vi "RTM CreateFramesSection.vi"(8 "error in (no error)":errorcluster, 10 "Frame":string="Tx FRAME ", 11 "Node Ptr":T1 format="%.0x") -> (0 "error out":errorcluster, 3 "Node Ptr 2":T1 format="%.0x")   [LabVIEW 2018, in "CAN Gateway System Explorer.lvlib"]
uses:
  CAN Gateway System Explorer.lvlib
  <vilib>/NI Veristand/Custom Device API/Custom Device Item Ref.ctl
  Types/FramesCluster.ctl
  <vilib>/NI Veristand/Custom Device API/Get Item Property (Variant).vi
  Shared/Constants.vi
  <vilib>/NI Veristand/Custom Device Tools/Custom Device Utility Library/NI VeriStand - Search for Item by Name.vi
  <vilib>/NI Veristand/Custom Device API/Custom Device API.lvlib
  Shared/CAN Gateway Shared.lvlib
  <vilib>/NI Veristand/Custom Device Tools/Custom Device Utility Library/Custom Device Utility Library.lvlib
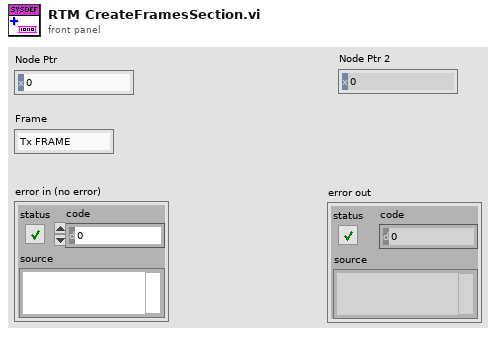
[diagram p1: front panel]
types:
  T1 = typedef "Custom Device API.lvlib/Custom Device Item Ref.ctl" = u64
  T2 = typedef "CAN Gateway System Explorer.lvlib/FramesCluster.ctl" = cluster{"Frame":string, "Fault":bool}
  T3 = typedef "Custom Device API.lvlib/Custom Device Item Info.ctl" = cluster{"Name":string, "Is Channel":bool, "GUID":string, "Is Waveform":bool}
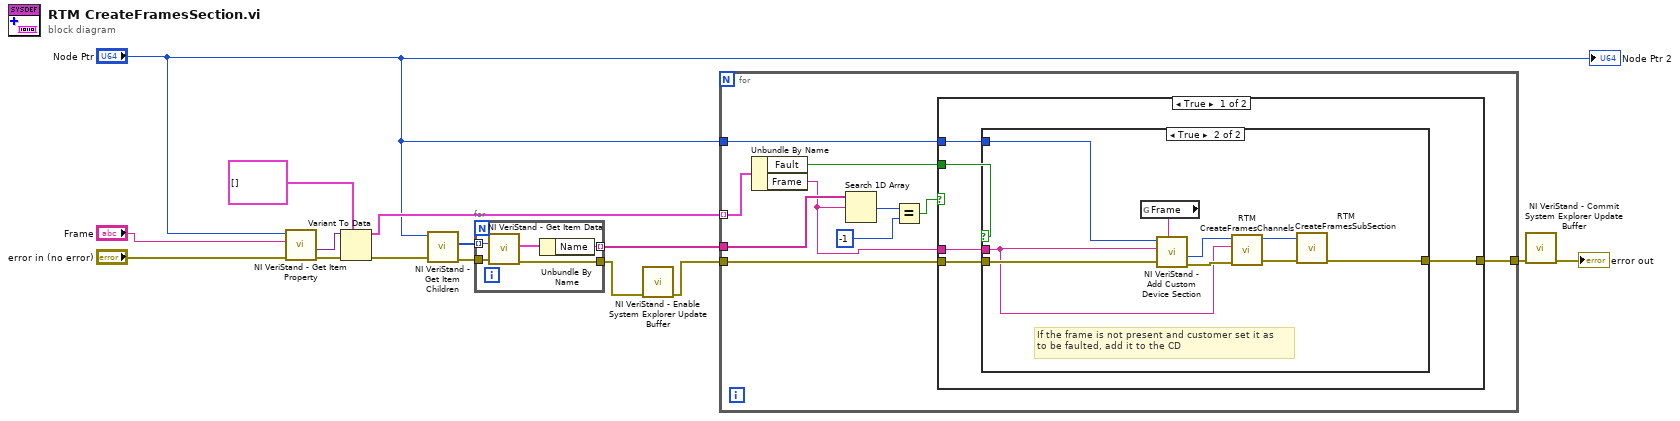
[diagram p0: block diagram]
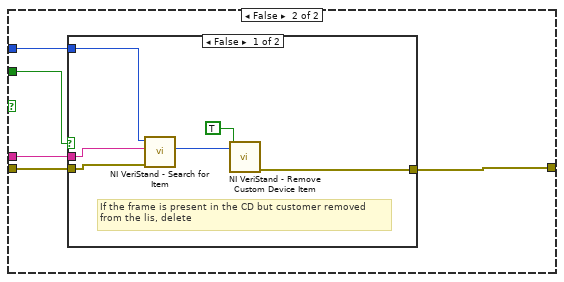
[diagram p3: hidden frame]
diagram:
  n1 = call-poly <vilib>:"NI VeriStand - Get Item Property.vi"("error in (no error)"="error in (no error)", "Property Name"="Frame", "Item Ref in"="Node Ptr") -> ("error out"=w14:errorcluster, "Value"=w15:variant)  [unwired: 5 in, 2 out]
  n2 = Variant To Data(error in=w14, type=T2[] [], Variant=w15) -> (data=w10:T2[], error out=w11:errorcluster)
  n3 = call <vilib>:"NI VeriStand - Get Item Children.vi"("error in (no error)"=w11, "Item Ref in"="Node Ptr") -> ("error out"=w7:errorcluster, "Child Refs"=w9:T1[])  [unwired: 6 in, 2 out]
  n4 = for {
    tunnel: w9 -> [w20] mode=indexing
    tunnel: [w18] -> w8 mode=indexing
    tunnel: w7 -> [w17]
    tunnel: [w16] -> w5
    n5 = call <vilib>:"NI VeriStand - Get Item Data.vi"("error in (no error)"=w17, "Item Ref in"=w20) -> ("error out"=w16:errorcluster, "Item Info"=w19:T3)  [unwired: 6 in, 2 out]
    n6 = Unbundle By Name(w19) -> ("Name"=w18:string)
  }
  n7 = call <vilib>:"NI VeriStand - Enable System Explorer Update Buffer.vi"("error in (no error)"=w5) -> ("error out"=w4:errorcluster)  [unwired: 10 in]
  n8 = for {
    tunnel: w10 -> [w30] mode=indexing
    tunnel: w8 -> [w29]
    tunnel: w4 -> [w26]
    tunnel: [w25] -> w3
    tunnel: "Node Ptr" -> [w21]
    n9 = Unbundle By Name(w30) -> ("Fault"=w23:bool, "Frame"=w22:string)
    n10 = Search 1D Array(1D array=w29, element=w22) -> (index of element=w27:i32)  [unwired: 1 in]
    n11 = Equal?(x=w27, y=-1 ("x")) -> (x = y?=w24:bool)
    n12 = case shown="True" w24 {
      tunnel: w26 -> [w35 w50]
      tunnel: [w34 w49] -> w25
      tunnel: w23 -> [w31 w46]
      tunnel: w22 -> [w33 w48]
      tunnel: w21 -> [w32 w47]
      frame True {
        n13 = case shown="True" w31 {
          tunnel: w35 -> [w36 w45]
          tunnel: [w36 w37] -> w34
          tunnel: w33 -> [_ w40]
          tunnel: w32 -> [_ w44]
          frame False {
          }
          frame True {
            # "If the frame is not present and customer set it as \nto be faulted, add it to the CD"
            n14 = global read "Constants.vi" "Frame"() -> (w43:string)
            n15 = call <vilib>:"NI VeriStand - Add Custom Device Section.vi"("GUID (Default Section)"=w43, "error in (no error)"=w45, "Section Name"=w40, "Parent Ref in"=w44) -> ("error out"=w42:errorcluster, "Section Ptr"=w41:T1)  [unwired: 4 in, 2 out]
            n16 = call "RTM CreateFramesChannels.vi"("error in (no error)"=w42, "Frame"=w40, "Node Ptr"=w41) -> ("error out"=w39:errorcluster, "Node Ptr 2"=w38:T1)  [unwired: 7 in]
            n17 = call "RTM CreateFramesSubSection.vi"("error in (no error)"=w39, "Node Ptr"=w38) -> ("error out"=w37:errorcluster)  [unwired: 8 in, 1 out]
          }
        }
      }
      frame False {
        n18 = case shown="False" w46 {
          tunnel: w50 -> [w55 w57]
          tunnel: [w56 w57] -> w49
          tunnel: w48 -> [w53 _]
          tunnel: w47 -> [w54 _]
          frame False {
            # "If the frame is present in the CD but customer removed\nfrom the lis, delete"
            n19 = call-poly <vilib>:"NI VeriStand - Search for Item.vi"("error in"=w55, "Item Name"=w53, "Section Ref in"=w54) -> ("Item Ref"=w52:T1)  [unwired: 5 in, 3 out]
            n20 = call <vilib>:"NI VeriStand - Remove Custom Device Item.vi"("Force Delete (F)"=TRUE, "Item Ref in"=w52) -> ("error out"=w56:errorcluster)  [unwired: 8 in, 1 out]
          }
          frame True {
          }
        }
      }
    }
  }
  n21 = call <vilib>:"NI VeriStand - Commit System Explorer Update Buffer.vi"("error in (no error)"=w3) -> ("error out"=→"error out":errorcluster)  [unwired: 10 in]
  "Node Ptr 2" <- "Node Ptr"
